vi "Last Ack Created Event.vi"(10 "Event":refnum<class "Event.lvclass">, 11 "Last Ack Created Event in":refnum<class "Last Ack Created Event.lvclass">) -> (3 "Last Ack Created Event out":refnum<class "Last Ack Created Event.lvclass">)   [LabVIEW 2021, in "jettl.lvlib" / "Last Ack Created Event Msg Strategy.lvlib" / "Last Ack Created Event.lvclass"]
uses:
  Last Ack Created Event.lvclass
  Event/Event.lvclass
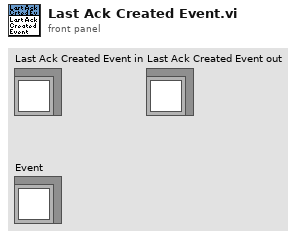
[diagram p1: front panel]
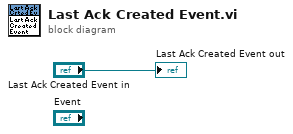
[diagram p0: block diagram]
diagram:
  "Last Ack Created Event out" <- "Last Ack Created Event in"
